vi "InitPython.vi"(8 "error in (no error)":errorcluster caption="entrée d'erreur (pas d'erreur)", 10 "Python Instruction":string, 11 "Scikit-learn en entrée":refnum<class "Scikit-learn.lvclass">) -> (0 "error out":errorcluster caption="sortie d'erreur", 3 "Scikit-learn en sortie":refnum<class "Scikit-learn.lvclass">)   [LabVIEW 2020, in "Scikit-learn.lvclass"]
doc: "Initialize session python"
uses:
  Scikit-learn.lvclass
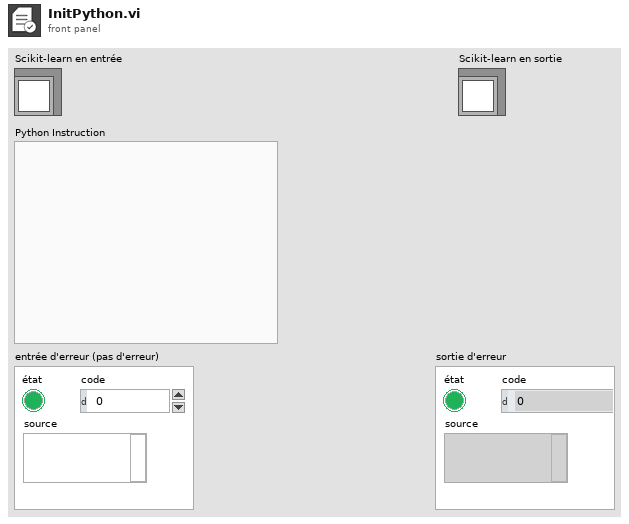
[diagram p1: front panel]
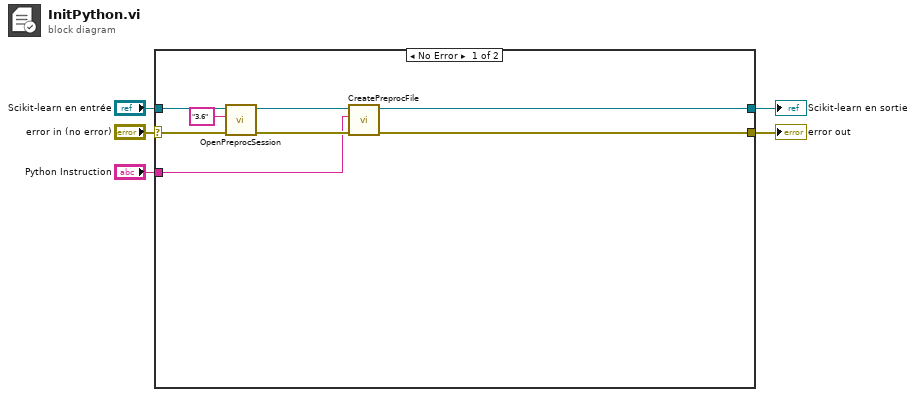
[diagram p0: block diagram]
diagram:
  n1 = case shown="No Error" "error in (no error)" {
    selector: "error in (no error)" -> [w7 w15]
    tunnel: [w8 w15] -> w4
    tunnel: [w9 w14] -> w2
    tunnel: "Scikit-learn en entrée" -> [w12 w14]
    tunnel: "Python Instruction" -> [w6 _]
    frame No Error {
      n2 = call-dynamic "OpenPreprocSession.vi"("error in (no error)"=w7, "Python version"="3.6", "Python in"=w12) -> ("error out"=w10:errorcluster, "Python out"=w11:refnum<class "Scikit-learn.lvclass">)  [unwired: 7 in]
      n3 = call-dynamic "CreatePreprocFile.vi"("error in (no error)"=w10, "Python Instruction"=w6, "Python in"=w11) -> ("error out"=w8:errorcluster, "Python out"=w9:refnum<class "Scikit-learn.lvclass">)  [unwired: 7 in]
    }
    frame Error {
    }
  }
  "error out" <- w4
  "Scikit-learn en sortie" <- w2
